vi "UART_Temperatura.vi"() -> ()   [LabVIEW 2020]
uses:
  <vilib>/Instr/_visa.llb/VISA Configure Serial Port (Instr).vi
panel:
  out "Boolean":bool
  in  "Numeric 5":dbl
  in  "Numeric 4":dbl
  out "Numeric 3":dbl
  out "Numeric 2":dbl
  out "Numeric":dbl
  out "Thermometer 2":dbl(slide) scale=0.0..1023.0
  out "Thermometer":dbl(slide) scale=0.0..1023.0
  in  "stop":bool
  out "String 2":string
  in  "VISA resource name":refnum<visa-resource-name>
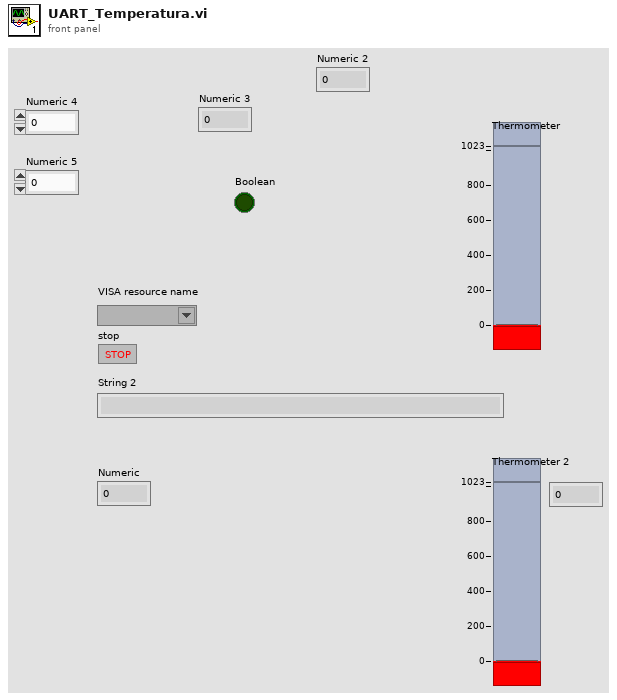
[diagram p1: front panel]
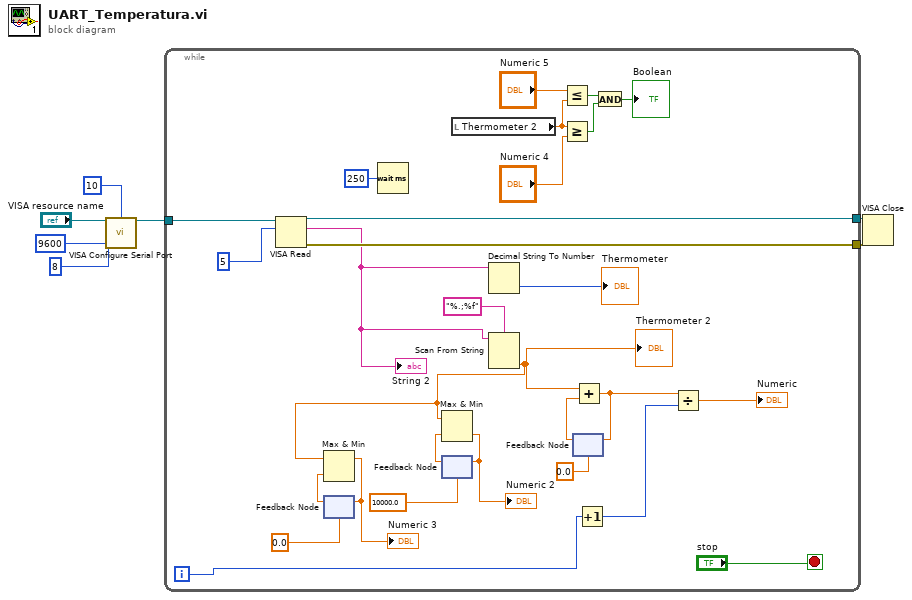
[diagram p0: block diagram]
diagram:
  n1 = call-poly "VISA Configure Serial Port"("VISA resource name"="VISA resource name", "termination char\n(0xA = '\\n' = LF)"=u8 10 ("termination char\n(0xA = '\\n' = LF)"), "baud rate (9600)"=u32 9600, "data bits (8)"=u16 8) -> ("VISA resource name out"=w4:refnum<visa-resource-name>)  [unwired: 10 in, 1 out]
  n2 = while {
    tunnel: w4 -> [w35]
    tunnel: [w32] -> w3
    tunnel: [w30] -> w2
    i -> [w22]
    stop <- "stop" stop-if-true
    n3 = VISA Read(VISA resource name=w35, byte count=u32 5) -> (VISA resource name out=w32:refnum<visa-resource-name>, read buffer=w27:string, error out=w30:errorcluster)  [unwired: 1 in, 1 out]
    "String 2" <- w27
    n4 = feedback #1(0.0) -> (w16:dbl)
    n5 = Wait (ms)(milliseconds to wait=u32 250) -> ()  [unwired: 1 out]
    n6 = feedback #2(10000.0) -> (w20:dbl)
    n7 = local read "Thermometer 2"() -> (w10:dbl)
    n8 = Decimal String To Number(string=w27) -> (number=→"Thermometer":i32)  [unwired: 2 in, 1 out]
    n9 = Scan From String(format string="%.;%f", input string=w27) -> (output 1=w14:dbl)  [unwired: 3 in, 3 out]
    "Thermometer 2" <- w14
    n10 = Max & Min(x=w14, y=w16) -> (max(x,y)=w15:dbl)  [unwired: 1 out]
    "Numeric 3" <- w15
    n11 = feedback-in #1(w15) -> ()
    n12 = Max & Min(x=w14, y=w20) -> (min(x,y)=w19:dbl)  [unwired: 1 out]
    "Numeric 2" <- w19
    n13 = feedback-in #2(w19) -> ()
    n14 = Less Or Equal?(x="Numeric 5", y=w10) -> (x <= y?=w11:bool)
    n15 = Greater Or Equal?(x=w10, y="Numeric 4") -> (x >= y?=w8:bool)
    n16 = feedback #3(0.0) -> (w26:dbl)
    n17 = Add(x=w14, y=w26) -> (x+y=w24:dbl)
    n18 = feedback-in #3(w24) -> ()
    n19 = Increment(x=w22) -> (x+1=w23:i32)
    n20 = And(x=w11, y=w8) -> (x .and. y?=→"Boolean":bool)
    n21 = Divide(x=w24, y=w23) -> (x/y=→"Numeric":dbl)
  }
  n22 = VISA Close(VISA resource name=w3, error in (no error)=w2) -> ()  [unwired: 1 out]
